vi "Build_Exe.vi"(8 "error in (no error)":errorcluster, 9 "Build Specification Version":T1, 10 "Workspace path":path, 11 "String in":refnum<vi>) -> (0 "error out":errorcluster)   [LabVIEW 2017]
uses:
  <vilib>/AppBuilder/AB_API_Simple/Build Specification Version.ctl
  BuildItem.ctl
  <vilib>/AppBuilder/AB_API_Simple/NI_App_Builder_API.lvlib
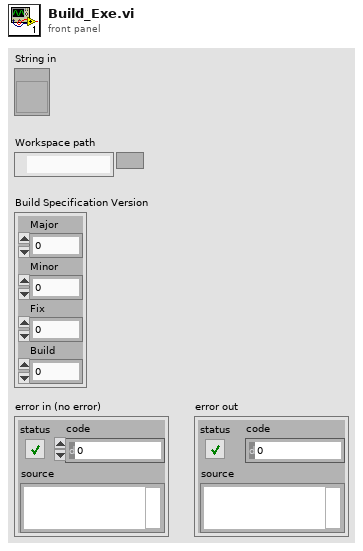
[diagram p1: front panel]
types:
  T1 = typedef "NI_App_Builder_API.lvlib/Build Specification Version.ctl" = cluster{"Major":u16, "Minor":u16, "Fix":u16, "Build":u16}
  T2 = typedef "BuildItem.ctl" = cluster{"Project":path, "BuildSpecification":path, "Destination":path}
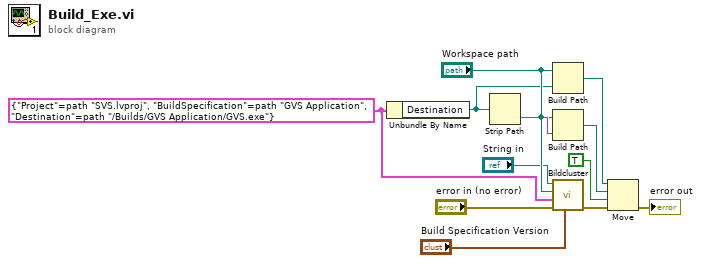
[diagram p0: block diagram]
diagram:
  w6 = T2 {"Project"=path "SVS.lvproj", "BuildSpecification"=path "GVS Application", "Destination"=path "../Builds/GVS Application/GVS.exe"} ("BuildItem")
  n1 = Unbundle By Name(w6) -> ("Destination"=w7:path)
  n2 = Strip Path(path=w7) -> (name=w9:string)  [unwired: 1 out]
  n3 = Build Path(base path="Workspace path", name or relative path=w7) -> (appended path=w2:path)
  n4 = Build Path(base path="Workspace path", name or relative path=w9) -> (appended path=w10:path)
  n5 = call "Bildcluster.vi"("Build Specification Version"="Build Specification Version", "error in (no error)"="error in (no error)", "BuildItem"=w6, "path"="Workspace path", "String in"="String in") -> ("error out"=w11:errorcluster)  [unwired: 6 in]
  n6 = Move(source path=w2, error in=w11, 9:TRUE ("overwrite (F)"), 10:w10) -> (error out=→"error out":errorcluster)  [unwired: 1 in, 2 out]
